vi "Callback - New Workbook.vi"(4 "User Parameter":variant, 5 "Event data":cluster{"Wb":refnum<k7>}, 6 "CtlRef":refnum<k7>, 7 "Event common data":cluster{"Source":i32, "Type":u32, "Time":u32}) -> ()   [LabVIEW 2023]
doc: "This callback VI runs whenever a new workbook is created in the Excel application."
panel:
  in  "Days of the Week":string[](array[string])=["Sunday", "Monday", "Tuesday", "Wednesday", "Thursday", "Friday", "Saturday"]
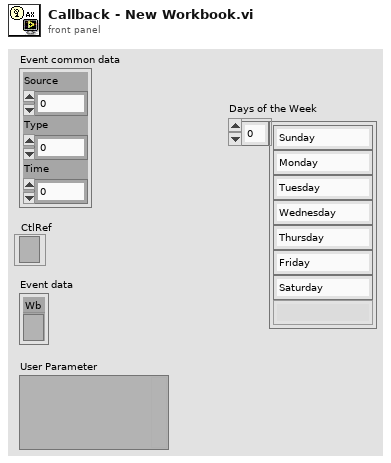
[diagram p1: front panel]
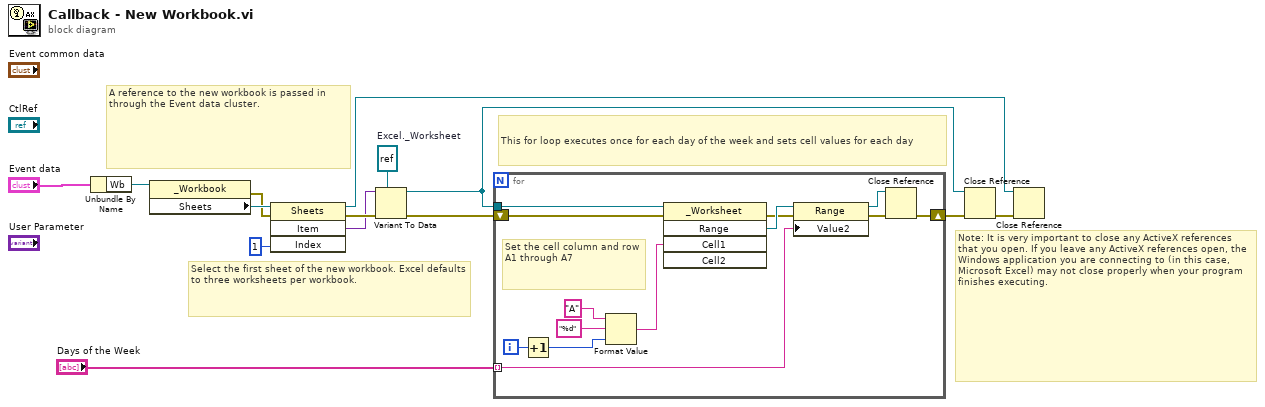
[diagram p0: block diagram]
diagram:
  w9 = refnum<k7> refnum  # Excel._Worksheet
  # "Note: It is very important to close any ActiveX references that you open. If you leave any ActiveX references open, the Windows application you are connecting to (in this case, Microsoft Excel) may not close properly when your program finishes executing."
  # "A reference to the new workbook is passed in through the Event data cluster."
  # "Select the first sheet of the new workbook. Excel defaults to three worksheets per workbook."
  # "This for loop executes once for each day of the week and sets cell values for each day"
  n1 = Unbundle By Name("Event data") -> ("Wb"=w6:refnum<k7>)
  n2 = property class="_Workbook"(reference=w6) -> (error out=w11:errorcluster, "Sheets"=w12:refnum<k7>)  [unwired: 1 in, 1 out]
  n3 = invoke class="Sheets" method="Item"(reference=w12, error in=w11, "Index"=1) -> (reference out=w1:refnum<k7>, error out=w8:errorcluster, "Item"=w7:variant)  [unwired: 1 in, 1 out]
  n4 = Variant To Data(error in=w8, type=w9, Variant=w7) -> (data=w3:refnum<k7>, error out=w14:errorcluster)
  n5 = for {
    tunnel: "Days of the Week" -> [w20] mode=indexing
    tunnel: w3 -> [w19]
    shift-right: [w16] -> w4
    shift-left: w14 -> [w18]
    i -> [w22]
    # "Set the cell column and row A1 through A7"
    n6 = Increment(x=w22) -> (x+1=w25:i32)
    n7 = Format Value(string ("")="A", format string="%d", value (0)=w25) -> (output string=w21:string)
    n8 = invoke class="_Worksheet" method="Range"(reference=w19, error in=w18, "Cell1"=w21) -> (error out=w26:errorcluster, "Range"=w27:refnum<k7>)  [unwired: 2 in, 3 out]
    n9 = property class="Range"(reference=w27, error in=w26, "Value2"=w20) -> (reference out=w15:refnum<k7>, error out=w17:errorcluster)
    n10 = Close Reference(reference=w15, error in (no error)=w17) -> (error out=w16:errorcluster)
  }
  n11 = Close Reference(reference=w3, error in (no error)=w4) -> (error out=w2:errorcluster)
  n12 = Close Reference(reference=w1, error in (no error)=w2) -> ()  [unwired: 1 out]
